vi "Not In Unified Msg Set.vi"(11 "Core Actor in":refnum<class "Core Actor.lvclass">) -> (0 "Error out":errorcluster, 3 "Core Actor out":refnum<class "Core Actor.lvclass">)   [LabVIEW 2025, in "jettl.lvlib" / "Actor.lvlib" / "Core Actor.lvclass"]
uses:
  Core Actor.lvclass
  Core Actor.lvclass/Core Actor.ctl
  Error/Error.lvlib
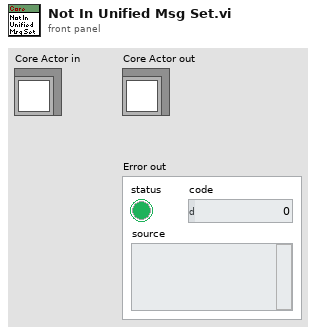
[diagram p1: front panel]
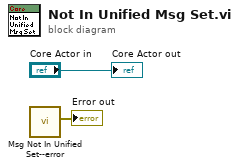
[diagram p0: block diagram]
diagram:
  n1 = call "Msg Not In Unified Set--error.vi"() -> ("Error"=→"Error out":errorcluster)  [unwired: 11 in]
  "Core Actor out" <- "Core Actor in"
